vi "Configure Internal Sweep Trigger.vi"(0 "VISA resource name":refnum<visa-resource-name>, 1 "External Trigger Source (0: Trigger1)":i32(ring) items=["Trigger1", "Trigger2", "Pulse"], 2 "Trigger Slope (0: Positive)":i32(ring) items=["Positive", "Negative"], 5 "Modulation Type (0: Amplitude Modulation)":i32(ring) items=["Amplitude Modulation", "Frequency Modulation", "Phase Modulation", "Low Frequency Output"], 7 "Modulation Path (1: 1)":i32(ring)=1 items=["1"=1, "2"=2], 9 "Trigger Source (1: Immediate)":i32(ring)=1 items=["Bus", "Immediate", "External", "Internal", "Key"], 11 "error in (no error)":errorcluster, 12 "Internal Trigger Source (0: Pulse Video)":i32(ring) items=["Pulse Video", "Pulse Sync"]) -> (4 "VISA resource name out":refnum<visa-resource-name>, 15 "error out":errorcluster)   [LabVIEW 2014, in "Agilent PSG MXG Series.lvlib"]
doc: "Configures trigger for internal sweep.\n\n<B>Notes:</B>\n(1) This VI is valid only inN5171B, N5172B, N5181B, N5182B that install <B>Option UNT</B> and <B>Option 303</B> (AM, FM, phase modulation, and LF output)."
uses:
  Agilent PSG MXG Series.lvlib
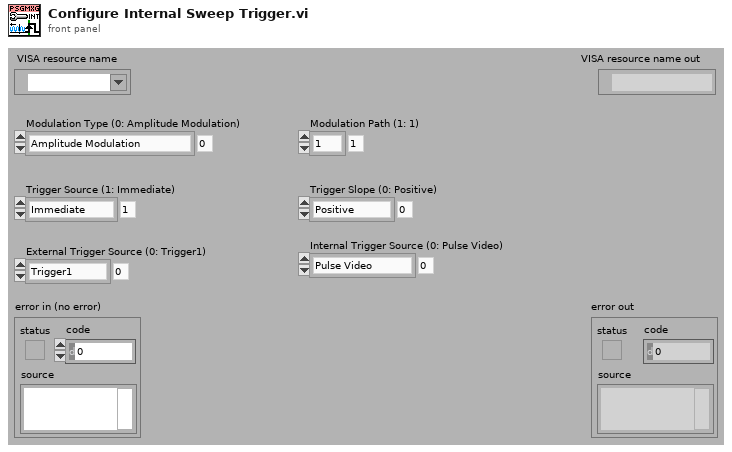
[diagram p1: front panel]
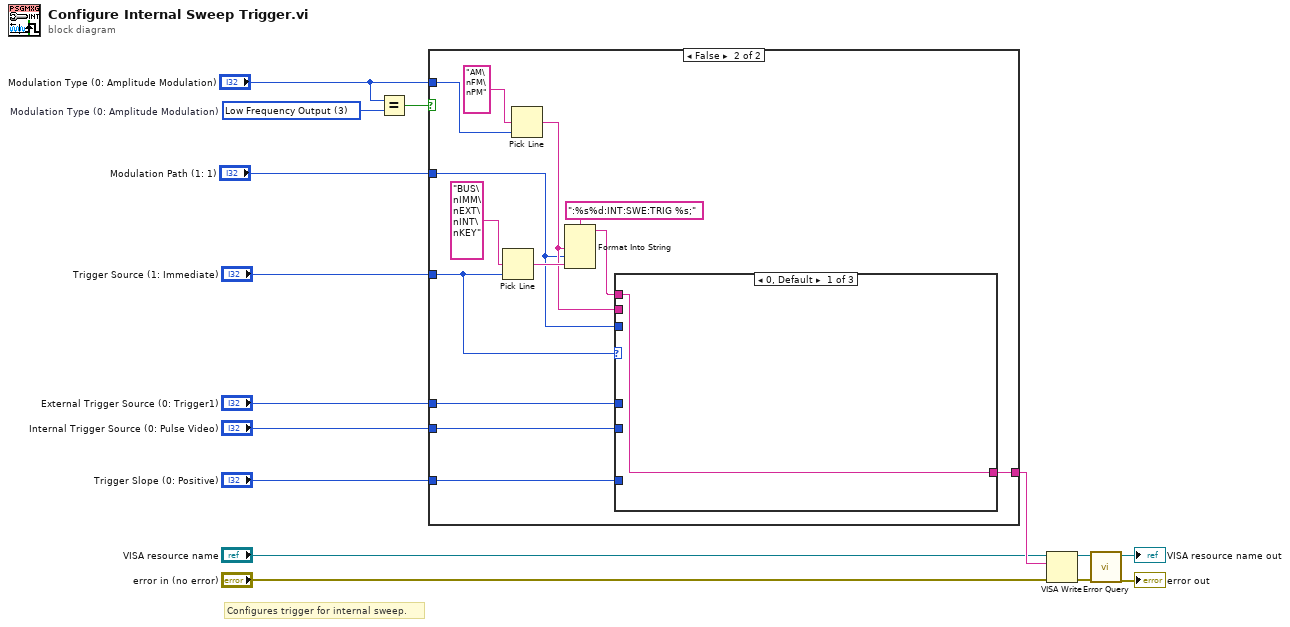
[diagram p0: block diagram]
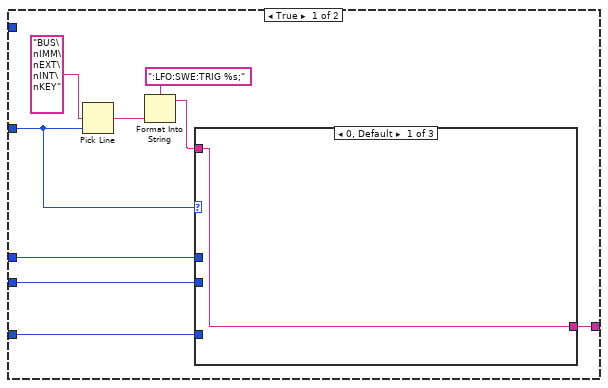
[diagram p2: hidden frame]
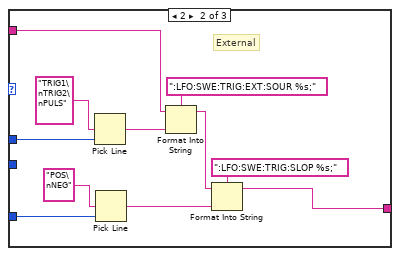
[diagram p3: hidden frame]
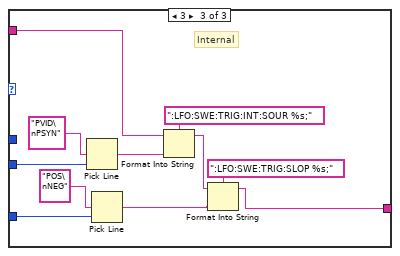
[diagram p4: hidden frame]
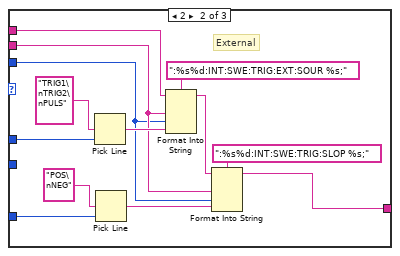
[diagram p5: hidden frame]
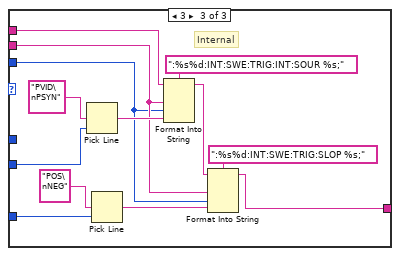
[diagram p6: hidden frame]
diagram:
  w3 = 3 items=["Amplitude Modulation", "Frequency Modulation", "Phase Modulation", "Low Frequency Output"]  # Modulation Type (0: Amplitude Modulation)
  # "Configures trigger for internal sweep."
  n1 = Equal?(x="Modulation Type (0: Amplitude Modulation)", y=w3) -> (x = y?=w4:bool)
  n2 = case shown="False" w4 {
    tunnel: "Trigger Source (1: Immediate)" -> [w19 w52]
    tunnel: "External Trigger Source (0: Trigger1)" -> [w22 w58]
    tunnel: "Internal Trigger Source (0: Pulse Video)" -> [w17 w48]
    tunnel: "Trigger Slope (0: Positive)" -> [w21 w57]
    tunnel: [w20 w56] -> w11
    tunnel: "Modulation Type (0: Amplitude Modulation)" -> [_ w54]
    tunnel: "Modulation Path (1: 1)" -> [_ w50]
    frame True {
      n3 = Pick Line(multi-line string="BUS\nIMM\nEXT\nINT\nKEY", line index=w19) -> (output string=w16:string)  [unwired: 1 out]
      n4 = Format Into String(format string=":LFO:SWE:TRIG %s;", w16) -> (resulting string=w18:string)  [unwired: 2 in, 1 out]
      n5 = case shown="0, Default" w19 {
        tunnel: w22 -> [_ w35 _]
        tunnel: w21 -> [_ w32 w43]
        tunnel: [w25 w30 w42] -> w20
        tunnel: w18 -> [w25 w29 w45]
        tunnel: w17 -> [_ _ w38]
        frame 0, Default {
        }
        frame 2 {
          # "External"
          n6 = Pick Line(multi-line string="TRIG1\nTRIG2\nPULS", line index=w35) -> (output string=w27:string)  [unwired: 1 out]
          n7 = Pick Line(multi-line string="POS\nNEG", line index=w32) -> (output string=w26:string)  [unwired: 1 out]
          n8 = Format Into String(format string=":LFO:SWE:TRIG:EXT:SOUR %s;", initial string=w29, w27) -> (resulting string=w28:string)  [unwired: 1 in, 1 out]
          n9 = Format Into String(format string=":LFO:SWE:TRIG:SLOP %s;", initial string=w28, w26) -> (resulting string=w30:string)  [unwired: 1 in, 1 out]
        }
        frame 3 {
          # "Internal"
          n10 = Pick Line(multi-line string="PVID\nPSYN", line index=w38) -> (output string=w40:string)  [unwired: 1 out]
          n11 = Pick Line(multi-line string="POS\nNEG", line index=w43) -> (output string=w39:string)  [unwired: 1 out]
          n12 = Format Into String(format string=":LFO:SWE:TRIG:INT:SOUR %s;", initial string=w45, w40) -> (resulting string=w41:string)  [unwired: 1 in, 1 out]
          n13 = Format Into String(format string=":LFO:SWE:TRIG:SLOP %s;", initial string=w41, w39) -> (resulting string=w42:string)  [unwired: 1 in, 1 out]
        }
      }
    }
    frame False {
      n14 = Pick Line(multi-line string="BUS\nIMM\nEXT\nINT\nKEY", line index=w52) -> (output string=w53:string)  [unwired: 1 out]
      n15 = Pick Line(multi-line string="AM\nFM\nPM", line index=w54) -> (output string=w51:string)  [unwired: 1 out]
      n16 = Format Into String(format string=":%s%d:INT:SWE:TRIG %s;", w51, w50, w53) -> (resulting string=w49:string)  [unwired: 2 in, 1 out]
      n17 = case shown="0, Default" w52 {
        tunnel: w58 -> [_ w73 _]
        tunnel: w57 -> [_ w70 w81]
        tunnel: [w61 w68 w78] -> w56
        tunnel: w51 -> [_ w64 w80]
        tunnel: w50 -> [_ w63 w79]
        tunnel: w49 -> [w61 w66 w85]
        tunnel: w48 -> [_ _ w76]
        frame 0, Default {
        }
        frame 2 {
          # "External"
          n18 = Pick Line(multi-line string="TRIG1\nTRIG2\nPULS", line index=w73) -> (output string=w67:string)  [unwired: 1 out]
          n19 = Pick Line(multi-line string="POS\nNEG", line index=w70) -> (output string=w62:string)  [unwired: 1 out]
          n20 = Format Into String(format string=":%s%d:INT:SWE:TRIG:EXT:SOUR %s;", initial string=w66, w64, w63, w67) -> (resulting string=w65:string)  [unwired: 1 in, 1 out]
          n21 = Format Into String(format string=":%s%d:INT:SWE:TRIG:SLOP %s;", initial string=w65, w64, w63, w62) -> (resulting string=w68:string)  [unwired: 1 in, 1 out]
        }
        frame 3 {
          # "Internal"
          n22 = Pick Line(multi-line string="PVID\nPSYN", line index=w76) -> (output string=w84:string)  [unwired: 1 out]
          n23 = Pick Line(multi-line string="POS\nNEG", line index=w81) -> (output string=w83:string)  [unwired: 1 out]
          n24 = Format Into String(format string=":%s%d:INT:SWE:TRIG:INT:SOUR %s;", initial string=w85, w80, w79, w84) -> (resulting string=w77:string)  [unwired: 1 in, 1 out]
          n25 = Format Into String(format string=":%s%d:INT:SWE:TRIG:SLOP %s;", initial string=w77, w80, w79, w83) -> (resulting string=w78:string)  [unwired: 1 in, 1 out]
        }
      }
    }
  }
  n26 = VISA Write(VISA resource name="VISA resource name", write buffer=w11, error in (no error)="error in (no error)") -> (VISA resource name out=w8:refnum<visa-resource-name>, error out=w7:errorcluster)  [unwired: 1 out]
  n27 = call "Error Query.vi"("error in (no error)"=w7, "VISA resource name"=w8) -> ("error out"=→"error out":errorcluster, "VISA resource name out"=→"VISA resource name out":refnum<visa-resource-name>)  [unwired: 8 out]
